vi "Execute Pre-Buffer.vi"(9 "MP Name":string, 10 "PIDF Profile Slot Select":dbl) -> ()   [LabVIEW 2016]
uses:
  Global Variables/MotionProfile.vi
  <vilib>/Rock Robotics/Network Tables/NT Write String.vi
  Global Variables/Refnum Names.vi
  <vilib>/Utility/file.llb/Read Delimited Spreadsheet (DBL).vi
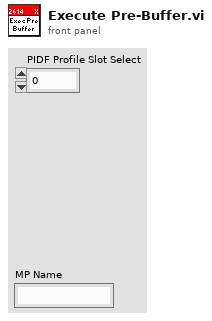
[diagram p1: front panel]
types:
  T1 = typedef "MotionProfile TypeDef.ctl" = cluster{"Left MP Array":dbl[][], "Left MP Index":dbl, "Semaphore":bool, "Right MP Array":dbl[][], "Right MP Index":dbl}
  T2 = typedef "WPI_MotorControlDeviceRef.ctl" = cluster{"DeviceStatus":errorcluster, "Type":T3, "PWM":cluster{"PWM Channel":T4, "DeadBand":T5}, "CAN":cluster{"Device Number":u8, "SetOutput VI Ref":variant, "GetOutput VI Ref":variant, "Enable VI Ref":variant, "Disable VI Ref":variant, "Data":variant}, "Invert":bool}
  T3 = typedef "WPI_MotorControlType.ctl" = enum16{"PWM", "CAN"}
  T4 = typedef "FPGA_DIOPWMChannel.ctl" = enum8{"PWM 0", "PWM 1", "PWM 2", "PWM 3", "PWM 4", "PWM 5", "PWM 6", "PWM 7", "PWM 8", "PWM 9", "PWM MXP 0", "PWM MXP 1", "PWM MXP 2", "PWM MXP 3", "PWM MXP 4", "PWM MXP 5", "PWM MXP 6", "PWM MXP 7", "PWM MXP 8", "PWM MXP 9", "Invalid"}
  T5 = typedef "WPI_PWMDeadband.ctl" = cluster{"Name":string, "maxPositivePwm":i32, "minPositivePwm":i32, "centerPwm":i32, "maxNegativePwm":i32, "minNegativePwm":i32, "angularRange":u16}
  T6 = typedef "WPI_CANTalonSRX_GlobalStatus.ctl" = cluster{"Applied Throttle":dbl, "Module Enabled":bool, "CAN Error":errorcluster, "Closed Loop Error":dbl, "Forward Limit Switch Closed":bool, "Reverse Limit Switch Closed":bool, "Sensor Position":dbl, "Sensor Velocity":dbl, "Current":dbl, "Sticky Fault - Over Temp":bool, "Sticky Fault - Under Voltage":bool, "Sticky Fault - Forward Limit":bool, "Sticky Fault - Reverse Limit":bool, "Sticky Fault - Forward Soft Limit":bool, "Sticky Fault - Reverse Soft Limit":bool, "Brake is Enabled":bool, "Encoder Position":dbl, "Encoder Velocity":dbl, "Encoder Index Count":dbl, "Encoder A Pin State":bool, "Encoder B Pin State":bool, "Encoder Index Pin State":bool, "Analog In":dbl, "Analog In Velocity":dbl, "Temperature (C)":dbl, "Battery Voltage":dbl, "Control 5 Is Supported":bool, "Current Profile Slot Select":dbl, "Pos Div 8":bool, "Vel Div 4":bool, "Pulse Width Position":i32, "Pulse Width Velocity":i32, "Pulse Width Rise To Rise (us)":i32, "Pulse Width Rise To Fall (us)":i32, "Mot Prof Active Is Under Run":bool, "Mot Prof Active Has Under Run":bool, "Mot Prof Active Is Last":bool, "Mot Prof Active Velocity Only":bool, "Mot Prof Active Is Valid":bool, "Mot Prof Buffer Is Full":bool, "Mot Prof Active Profile Slot Select":i32, "Mot Prof NextID":i32, "Mot Prof Count":i32, "Mot Prof Active Velocity":dbl, "Mot Prof Active Position":dbl, "Mot Prof Output Enable":i32, "UsageFrame":u32, "Motion Magic Active Trajectory":cluster{"Velocity":dbl, "Position":dbl}}
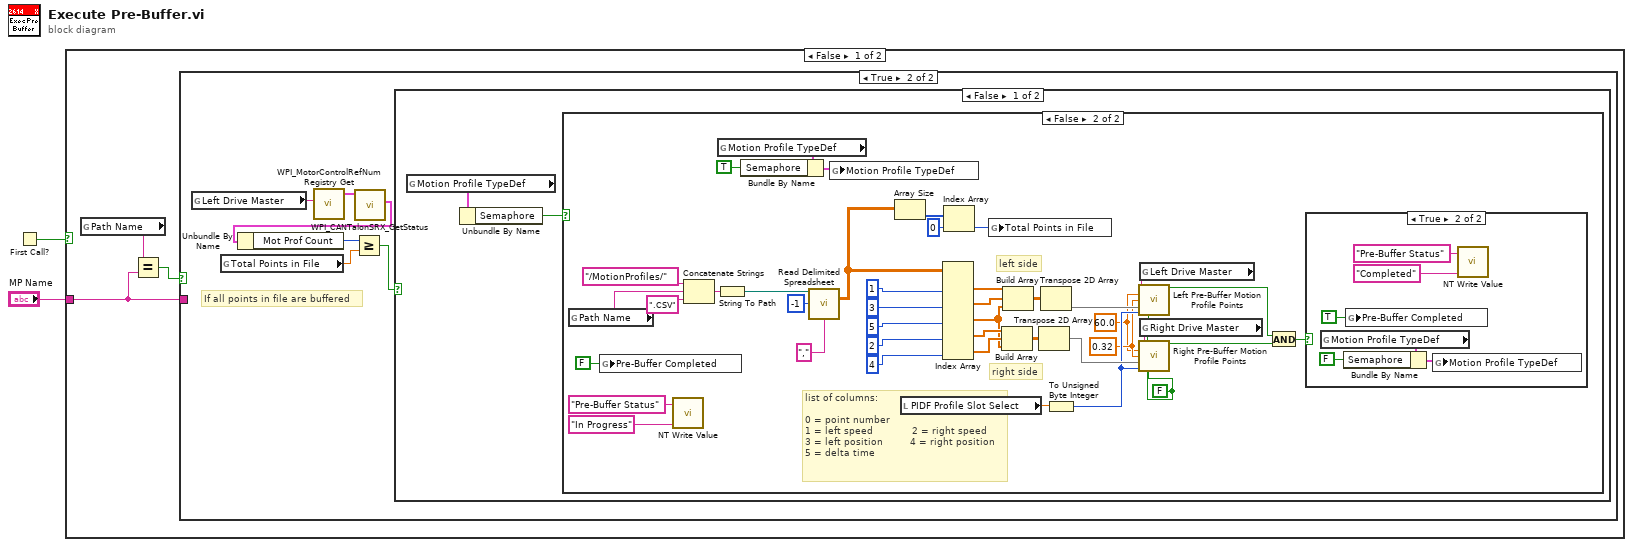
[diagram p0: block diagram]
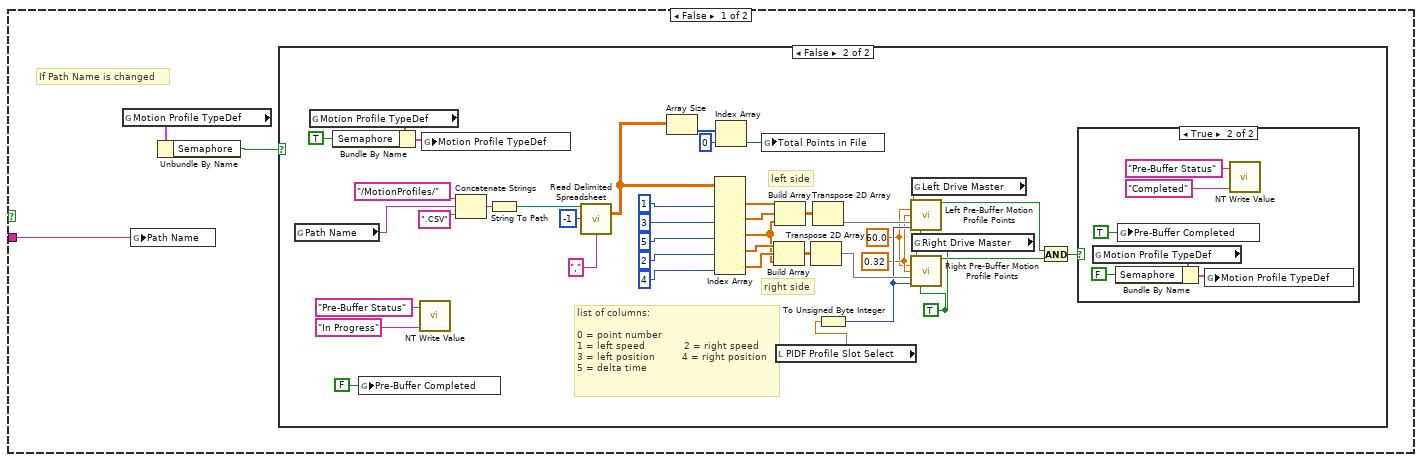
[diagram p2: hidden frame]
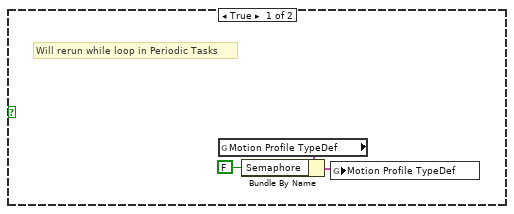
[diagram p3: hidden frame]
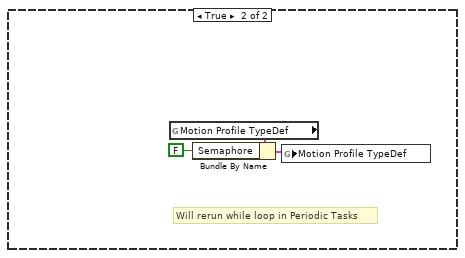
[diagram p7: hidden frame]
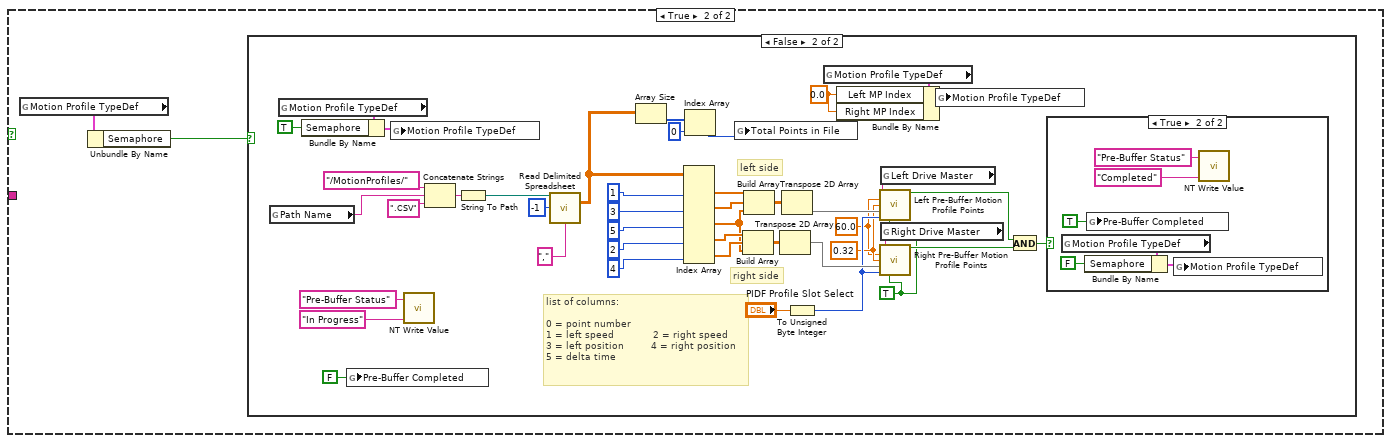
[diagram p8: hidden frame]
diagram:
  n1 = First Call?() -> (First Call?: T/F=w1:bool)
  n2 = case shown="False" w1 {
    tunnel: "MP Name" -> [w3 _]
    frame False {
      n3 = global read "MotionProfile.vi" "Path Name"() -> (w5:string)
      n4 = Equal?(x=w5, y=w3) -> (x = y?=w4:bool)
      n5 = case shown="True" w4 {
        tunnel: w3 -> [w8 _]
        frame False {
          # "If Path Name is changed"
          n6 = global read "MotionProfile.vi" "Motion Profile TypeDef"() -> (w7:T1)
          n7 = global write "MotionProfile.vi" "Path Name"(w8) -> ()
          n8 = Unbundle By Name(w7) -> ("Semaphore"=w6:bool)
          n9 = case shown="False" w6 {
            frame True {
              # "Will rerun while loop in Periodic Tasks"
              n10 = global read "MotionProfile.vi" "Motion Profile TypeDef"() -> (w11:T1)
              n11 = Bundle By Name(cluster=w11, "Semaphore"=FALSE) -> (w10:T1)
              n12 = global write "MotionProfile.vi" "Motion Profile TypeDef"(w10) -> ()
            }
            frame False {
              w17 = TRUE
              w19 = 60.0 ("Time Conversion Factor")
              w20 = 0.32 ("Linear Conversion Factor")
              # "list of columns:\n\n0 = point number\n1 = left speed             2 = right speed\n3 = left position         4 = right position\n5 = delta time"
              # "left side"
              # "right side"
              n13 = global read "MotionProfile.vi" "Path Name"() -> (w18:string)
              n14 = global read "MotionProfile.vi" "Motion Profile TypeDef"() -> (w26:T1)
              n15 = Bundle By Name(cluster=w26, "Semaphore"=TRUE) -> (w25:T1)
              n16 = global write "MotionProfile.vi" "Pre-Buffer Completed"(FALSE ("Pre-Buffer Completed")) -> ()
              n17 = call-poly <vilib>:"NT Write Value.vi"("String"="In Progress", "Name"="Pre-Buffer Status") -> ()  [unwired: 9 in, 1 out]
              n18 = global write "MotionProfile.vi" "Motion Profile TypeDef"(w25) -> ()
              n19 = Concatenate Strings("/MotionProfiles/" ("string"), w18, ".CSV" ("string")) -> (w50:string)
              n20 = String To Path(string=w50) -> (path=w47:path)
              n21 = call-poly <vilib>:"Read Delimited Spreadsheet.vi"("file path (dialog if empty)"=w47, "number of rows (all:-1)"=-1, "delimiter (\\t)"="," ("delimiter (\\t)")) -> ("all rows"=w33:dbl[][])  [unwired: 7 in, 5 out]
              n22 = Array Size(array=w33) -> (size(s)=w32:i32[])
              n23 = Index Array(array=w33, index (col) #1=1 ("disabled index (col)"), index (col) #2=3 ("disabled index (col)"), index (col) #3=5 ("disabled index (col)"), index (col) #4=2 ("disabled index (col)"), index (col) #5=4 ("disabled index (col)")) -> (element #1=w40:dbl[], element #2=w39:dbl[], element #3=w36:dbl[], element #4=w38:dbl[], element #5=w37:dbl[])  [unwired: 5 in]
              n24 = Index Array(array=w32, index=0) -> (element=w12:i32)
              n25 = global write "MotionProfile.vi" "Total Points in File"(w12) -> ()
              n26 = Build Array(w38, w37, w36) -> (w34:dbl[][])
              n27 = Build Array(w40, w39, w36) -> (w35:dbl[][])
              n28 = local read "PIDF Profile Slot Select"() -> (w16:dbl)
              n29 = Transpose 2D Array(2D array=w34) -> (transposed array=w28:dbl[][])
              n30 = Transpose 2D Array(2D array=w35) -> (transposed array=w29:dbl[][])
              n31 = To Unsigned Byte Integer(number=w16) -> (unsigned 8bit integer=w27:u8)
              n32 = global read "Refnum Names.vi" "Left Drive Master"() -> (w31:string)
              n33 = call "Left Pre-Buffer Motion Profile Points.vi"("Motor Name"=w31, "Time Conversion Factor"=w19, "Linear Conversion Factor"=w20, "Motion Profile Array"=w29, "PIDF Profile Slot Select"=w27, "Clear Buffer"=w17) -> ("Ready to Execute"=w23:bool)  [unwired: 9 in]
              n34 = global read "Refnum Names.vi" "Right Drive Master"() -> (w30:string)
              n35 = call "Right Pre-Buffer Motion Profile Points.vi"("Motor Name"=w30, "Time Conversion Factor"=w19, "Linear Conversion Factor"=w20, "Motion Profile Array"=w28, "PIDF Profile Slot Select"=w27, "Clear Buffer"=w17) -> ("Ready to Execute"=w22:bool)  [unwired: 9 in]
              n36 = And(x=w23, y=w22) -> (x .and. y?=w21:bool)
              n37 = case shown="True" w21 {
                frame False {
                }
                frame True {
                  n38 = global read "MotionProfile.vi" "Motion Profile TypeDef"() -> (w58:T1)
                  n39 = Bundle By Name(cluster=w58, "Semaphore"=FALSE) -> (w57:T1)
                  n40 = global write "MotionProfile.vi" "Pre-Buffer Completed"(TRUE ("Pre-Buffer Completed")) -> ()
                  n41 = global write "MotionProfile.vi" "Motion Profile TypeDef"(w57) -> ()
                  n42 = call-poly <vilib>:"NT Write Value.vi"("String"="Completed", "Name"="Pre-Buffer Status") -> ()  [unwired: 9 in, 1 out]
                }
              }
            }
          }
        }
        frame True {
          # "If all points in file are buffered"
          n43 = global read "Refnum Names.vi" "Left Drive Master"() -> (w64:string)
          n44 = global read "MotionProfile.vi" "Total Points in File"() -> (w59:dbl)
          n45 = call <vilib>:"WPI_MotorControlRefNum Registry Get.vi"("refnum name"=w64) -> ("MotorControlDevRef"=w62:T2)  [unwired: 9 in, 1 out]
          n46 = call <vilib>:"WPI_CANTalonSRX_GetStatus.vi"("CAN Talon SRX Ref"=w62) -> ("Talon SRX Status"=w61:T6)  [unwired: 8 in, 2 out]
          n47 = Unbundle By Name(w61) -> ("Mot Prof Count"=w60:i32)
          n48 = Greater Or Equal?(x=w60, y=w59) -> (x >= y?=w63:bool)
          n49 = case shown="False" w63 {
            frame False {
              n50 = global read "MotionProfile.vi" "Motion Profile TypeDef"() -> (w66:T1)
              n51 = Unbundle By Name(w66) -> ("Semaphore"=w65:bool)
              n52 = case shown="False" w65 {
                frame True {
                  # "Will rerun while loop in Periodic Tasks"
                }
                frame False {
                  w72 = FALSE
                  w74 = 60.0 ("Time Conversion Factor")
                  w75 = 0.32 ("Linear Conversion Factor")
                  # "list of columns:\n\n0 = point number\n1 = left speed             2 = right speed\n3 = left position         4 = right position\n5 = delta time"
                  # "left side"
                  # "right side"
                  n53 = global read "MotionProfile.vi" "Path Name"() -> (w73:string)
                  n54 = global write "MotionProfile.vi" "Pre-Buffer Completed"(FALSE ("Pre-Buffer Completed")) -> ()
                  n55 = call-poly <vilib>:"NT Write Value.vi"("String"="In Progress", "Name"="Pre-Buffer Status") -> ()  [unwired: 9 in, 1 out]
                  n56 = Concatenate Strings("/MotionProfiles/" ("string"), w73, ".CSV" ("string")) -> (w105:string)
                  n57 = String To Path(string=w105) -> (path=w102:path)
                  n58 = global read "MotionProfile.vi" "Motion Profile TypeDef"() -> (w81:T1)
                  n59 = Bundle By Name(cluster=w81, "Semaphore"=TRUE) -> (w80:T1)
                  n60 = call-poly <vilib>:"Read Delimited Spreadsheet.vi"("file path (dialog if empty)"=w102, "number of rows (all:-1)"=-1, "delimiter (\\t)"="," ("delimiter (\\t)")) -> ("all rows"=w88:dbl[][])  [unwired: 7 in, 5 out]
                  n61 = global write "MotionProfile.vi" "Motion Profile TypeDef"(w80) -> ()
                  n62 = Array Size(array=w88) -> (size(s)=w87:i32[])
                  n63 = local read "PIDF Profile Slot Select"() -> (w71:dbl)
                  n64 = Index Array(array=w88, index (col) #1=1 ("disabled index (col)"), index (col) #2=3 ("disabled index (col)"), index (col) #3=5 ("disabled index (col)"), index (col) #4=2 ("disabled index (col)"), index (col) #5=4 ("disabled index (col)")) -> (element #1=w95:dbl[], element #2=w94:dbl[], element #3=w91:dbl[], element #4=w93:dbl[], element #5=w92:dbl[])  [unwired: 5 in]
                  n65 = Index Array(array=w87, index=0) -> (element=w67:i32)
                  n66 = global write "MotionProfile.vi" "Total Points in File"(w67) -> ()
                  n67 = Build Array(w93, w92, w91) -> (w89:dbl[][])
                  n68 = Build Array(w95, w94, w91) -> (w90:dbl[][])
                  n69 = Transpose 2D Array(2D array=w89) -> (transposed array=w83:dbl[][])
                  n70 = Transpose 2D Array(2D array=w90) -> (transposed array=w84:dbl[][])
                  n71 = To Unsigned Byte Integer(number=w71) -> (unsigned 8bit integer=w82:u8)
                  n72 = global read "Refnum Names.vi" "Left Drive Master"() -> (w86:string)
                  n73 = call "Left Pre-Buffer Motion Profile Points.vi"("Motor Name"=w86, "Time Conversion Factor"=w74, "Linear Conversion Factor"=w75, "Motion Profile Array"=w84, "PIDF Profile Slot Select"=w82, "Clear Buffer"=w72) -> ("Ready to Execute"=w78:bool)  [unwired: 9 in]
                  n74 = global read "Refnum Names.vi" "Right Drive Master"() -> (w85:string)
                  n75 = call "Right Pre-Buffer Motion Profile Points.vi"("Motor Name"=w85, "Time Conversion Factor"=w74, "Linear Conversion Factor"=w75, "Motion Profile Array"=w83, "PIDF Profile Slot Select"=w82, "Clear Buffer"=w72) -> ("Ready to Execute"=w77:bool)  [unwired: 9 in]
                  n76 = And(x=w78, y=w77) -> (x .and. y?=w76:bool)
                  n77 = case shown="True" w76 {
                    frame False {
                    }
                    frame True {
                      n78 = global read "MotionProfile.vi" "Motion Profile TypeDef"() -> (w113:T1)
                      n79 = Bundle By Name(cluster=w113, "Semaphore"=FALSE) -> (w112:T1)
                      n80 = global write "MotionProfile.vi" "Pre-Buffer Completed"(TRUE ("Pre-Buffer Completed")) -> ()
                      n81 = global write "MotionProfile.vi" "Motion Profile TypeDef"(w112) -> ()
                      n82 = call-poly <vilib>:"NT Write Value.vi"("String"="Completed", "Name"="Pre-Buffer Status") -> ()  [unwired: 9 in, 1 out]
                    }
                  }
                }
              }
            }
            frame True {
              # "Will rerun while loop in Periodic Tasks"
              n83 = global read "MotionProfile.vi" "Motion Profile TypeDef"() -> (w114:T1)
              n84 = Bundle By Name(cluster=w114, "Semaphore"=FALSE) -> (w115:T1)
              n85 = global write "MotionProfile.vi" "Motion Profile TypeDef"(w115) -> ()
            }
          }
        }
      }
    }
    frame True {
      n86 = global read "MotionProfile.vi" "Motion Profile TypeDef"() -> (w118:T1)
      n87 = Unbundle By Name(w118) -> ("Semaphore"=w117:bool)
      n88 = case shown="False" w117 {
        frame True {
          # "Will rerun while loop in Periodic Tasks"
        }
        frame False {
          w120 = 0.0 ("Left MP Index")
          w123 = TRUE
          w128 = 60.0 ("Time Conversion Factor")
          w129 = 0.32 ("Linear Conversion Factor")
          # "list of columns:\n\n0 = point number\n1 = left speed             2 = right speed\n3 = left position         4 = right position\n5 = delta time"
          # "left side"
          # "right side"
          n89 = global read "MotionProfile.vi" "Path Name"() -> (w127:string)
          n90 = global read "MotionProfile.vi" "Motion Profile TypeDef"() -> (w135:T1)
          n91 = Bundle By Name(cluster=w135, "Semaphore"=TRUE) -> (w134:T1)
          n92 = global write "MotionProfile.vi" "Pre-Buffer Completed"(FALSE ("Pre-Buffer Completed")) -> ()
          n93 = global write "MotionProfile.vi" "Motion Profile TypeDef"(w134) -> ()
          n94 = call-poly <vilib>:"NT Write Value.vi"("String"="In Progress", "Name"="Pre-Buffer Status") -> ()  [unwired: 9 in, 1 out]
          n95 = Concatenate Strings("/MotionProfiles/" ("string"), w127, ".CSV" ("string")) -> (w160:string)
          n96 = String To Path(string=w160) -> (path=w157:path)
          n97 = call-poly <vilib>:"Read Delimited Spreadsheet.vi"("file path (dialog if empty)"=w157, "number of rows (all:-1)"=-1, "delimiter (\\t)"="," ("delimiter (\\t)")) -> ("all rows"=w143:dbl[][])  [unwired: 7 in, 5 out]
          n98 = Array Size(array=w143) -> (size(s)=w142:i32[])
          n99 = Index Array(array=w143, index (col) #1=1 ("disabled index (col)"), index (col) #2=3 ("disabled index (col)"), index (col) #3=5 ("disabled index (col)"), index (col) #4=2 ("disabled index (col)"), index (col) #5=4 ("disabled index (col)")) -> (element #1=w150:dbl[], element #2=w149:dbl[], element #3=w146:dbl[], element #4=w148:dbl[], element #5=w147:dbl[])  [unwired: 5 in]
          n100 = Index Array(array=w142, index=0) -> (element=w119:i32)
          n101 = global write "MotionProfile.vi" "Total Points in File"(w119) -> ()
          n102 = Build Array(w148, w147, w146) -> (w144:dbl[][])
          n103 = Build Array(w150, w149, w146) -> (w145:dbl[][])
          n104 = Transpose 2D Array(2D array=w144) -> (transposed array=w137:dbl[][])
          n105 = Transpose 2D Array(2D array=w145) -> (transposed array=w138:dbl[][])
          n106 = To Unsigned Byte Integer(number="PIDF Profile Slot Select") -> (unsigned 8bit integer=w136:u8)
          n107 = global read "MotionProfile.vi" "Motion Profile TypeDef"() -> (w122:T1)
          n108 = Bundle By Name(cluster=w122, "Left MP Index"=w120, "Right MP Index"=w120) -> (w121:T1)
          n109 = global read "Refnum Names.vi" "Left Drive Master"() -> (w140:string)
          n110 = call "Left Pre-Buffer Motion Profile Points.vi"("Motor Name"=w140, "Time Conversion Factor"=w128, "Linear Conversion Factor"=w129, "Motion Profile Array"=w138, "PIDF Profile Slot Select"=w136, "Clear Buffer"=w123) -> ("Ready to Execute"=w132:bool)  [unwired: 9 in]
          n111 = global read "Refnum Names.vi" "Right Drive Master"() -> (w139:string)
          n112 = call "Right Pre-Buffer Motion Profile Points.vi"("Motor Name"=w139, "Time Conversion Factor"=w128, "Linear Conversion Factor"=w129, "Motion Profile Array"=w137, "PIDF Profile Slot Select"=w136, "Clear Buffer"=w123) -> ("Ready to Execute"=w131:bool)  [unwired: 9 in]
          n113 = global write "MotionProfile.vi" "Motion Profile TypeDef"(w121) -> ()
          n114 = And(x=w132, y=w131) -> (x .and. y?=w130:bool)
          n115 = case shown="True" w130 {
            frame False {
            }
            frame True {
              n116 = global read "MotionProfile.vi" "Motion Profile TypeDef"() -> (w168:T1)
              n117 = Bundle By Name(cluster=w168, "Semaphore"=FALSE) -> (w167:T1)
              n118 = global write "MotionProfile.vi" "Pre-Buffer Completed"(TRUE ("Pre-Buffer Completed")) -> ()
              n119 = global write "MotionProfile.vi" "Motion Profile TypeDef"(w167) -> ()
              n120 = call-poly <vilib>:"NT Write Value.vi"("String"="Completed", "Name"="Pre-Buffer Status") -> ()  [unwired: 9 in, 1 out]
            }
          }
        }
      }
    }
  }
